vi "Shooter Power to Speed.vi"(9 "Shooter Wheel/Gear Ratio":dbl, 10 "Shooter Maxiimum Speed (rpm)":dbl, 11 "Shooter Power (%)":dbl) -> (3 "Disc Speed":dbl)   [LabVIEW 2012]
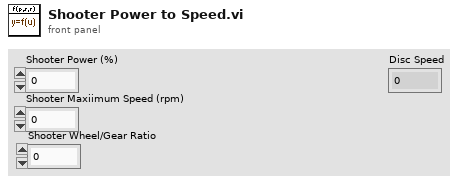
[diagram p1: front panel]
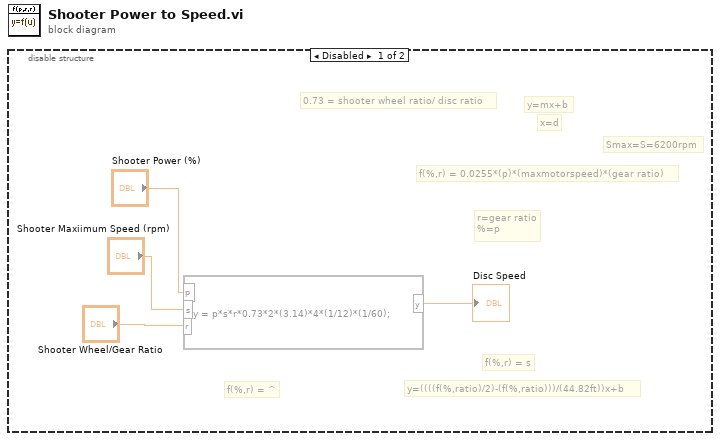
[diagram p0: block diagram]
diagram:
  n1 = disable-structure shown="Disabled" {
    frame Disabled {
      # "0.73 = shooter wheel ratio/ disc ratio"
      # "f(%,r) = ^"
      # "x=d"
      # "y=mx+b"
      # "Smax=S=6200rpm"
      # "f(%,r) = 0.0255*(p)*(maxmotorspeed)*(gear ratio)"
      # "r=gear ratio\n%=p"
      # "f(%,r) = s"
      # "y=((((f(%,ratio)/2)-(f(%,ratio)))/(44.82ft))x+b"
      n2 = formula code="y = p*s*r*0.73*2*(3.14)*4*(1/12)*(1/60);"("p"="Shooter Power (%)", "r"="Shooter Wheel/Gear Ratio", "s"="Shooter Maxiimum Speed (rpm)") -> ("y"=→"Disc Speed":dbl)
    }
    frame Enabled {
    }
  }
